vi "Anode State Cluster to Map.vi"(10 "Fmeasure (F, P1, P2) in":T1) -> (1 "Anode Status Map":map{string, dbl}(c390))   [LabVIEW 2024, in "Anode.lvlib"]
uses:
  Anode.lvlib
  Modbus Flexi-Flow API/Fmeasure (F,P1,P2)--cluster.ctl
  Modbus Flexi-Flow API/Bronkhorst Flexi-Flow ModbusTCP API.lvlib
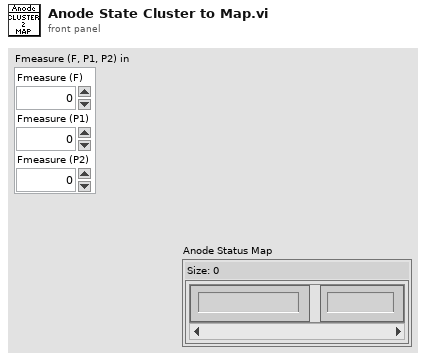
[diagram p1: front panel]
types:
  T1 = typedef "Bronkhorst Flexi-Flow ModbusTCP API.lvlib/Fmeasure (F,P1,P2)--cluster.ctl" = cluster{"Fmeasure (F)":sgl, "Fmeasure (P1)":sgl, "Fmeasure (P2)":sgl}
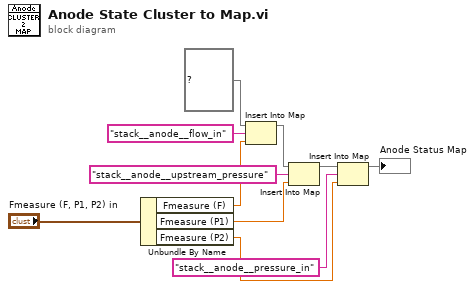
[diagram p0: block diagram]
diagram:
  n1 = Unbundle By Name("Fmeasure (F, P1, P2) in") -> ("Fmeasure (F)"=w7:sgl, "Fmeasure (P1)"=w6:sgl, "Fmeasure (P2)"=w5:sgl)
  n2 = Insert Into Map(map in=map{string, dbl} {} ("Anode Status Map"), key="stack__anode__flow_in", value=w7) -> (map out=w11:map{string, dbl})  [unwired: 2 out]
  n3 = Insert Into Map(map in=w11, key="stack__anode__upstream_pressure", value=w6) -> (map out=w10:map{string, dbl})  [unwired: 2 out]
  n4 = Insert Into Map(map in=w10, key="stack__anode__pressure_in", value=w5) -> (map out=→"Anode Status Map":map{string, dbl})  [unwired: 2 out]
